vi "Chrg_Dschrg_No_cDAQ0.vi"(0 "file path (use dialog)":path, 4 "PS VISA in":refnum<visa-resource-name>, 5 "PS error in":errorcluster, 6 "DischargeCyclePath":path=path "C:/Users/ga11/Desktop/VI/results/3PtestCharge.lvm" caption="Filename", 8 "Charge/discharge":enum8{"Charge", "Discharge"}(ring), 9 "Charge/Discharge Voltage Setpoint":dbl format="%#.6g", 10 "CC or CCCV":enum16{"CC", "CCCV"}(ring), 11 "Current Setpoint":dbl format="%#.6g", 12 "Output Safety":T1, 13 "Current Cutoff":dbl) -> (18 "PS VIS resource name out":refnum<visa-resource-name>, 19 "PS error out":errorcluster)   [LabVIEW 2020]
uses:
  Drivers-Essentials/global stop1.vi
  Drivers-NHR-9200/NHR/Public/Data/Low Level/Fetch (Ave Voltage).vi
  Drivers-NHR-9200/NHR/NH Research Regenerative Test Series.lvlib
panel:
  out "error out":errorcluster
  out "Read Ave Current (A)":dbl
  out "Read Ave Voltage (V)":dbl
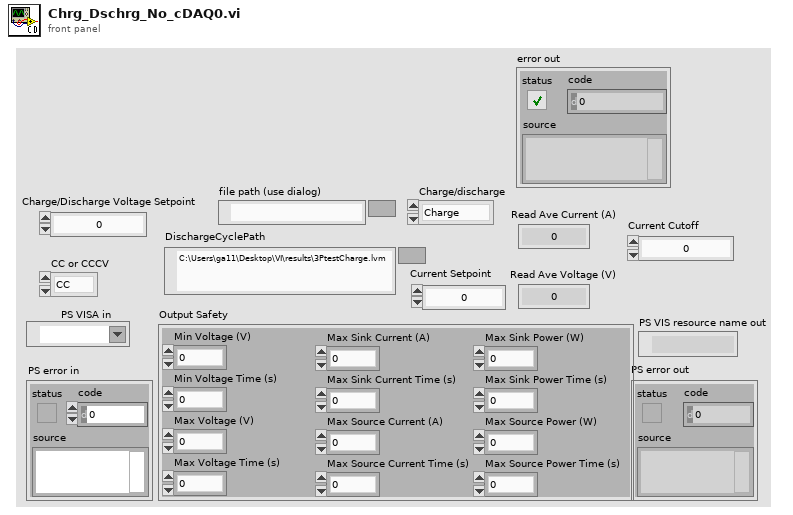
[diagram p1: front panel]
types:
  T1 = cluster{"Min Voltage (V)":dbl, "Min Voltage Time (s)":dbl, "Max Voltage (V)":dbl, "Max Voltage Time (s)":dbl, "Max Sink Current (A)":dbl, "Max Sink Current Time (s)":dbl, "Max Source Current (A)":dbl, "Max Source Current Time (s)":dbl, "Max Sink Power (W)":dbl, "Max Sink Power Time (s)":dbl, "Max Source Power (W)":dbl, "Max Source Power Time (s)":dbl}
  T2 = enum16{"open", "replace", "create", "open or create", "replace or create", "replace or create with confirmation"}
  T3 = cluster{"Voltage Enabled":bool, "Current Enabled":bool, "Power Enabled":bool, "Resistance Enabled":bool}
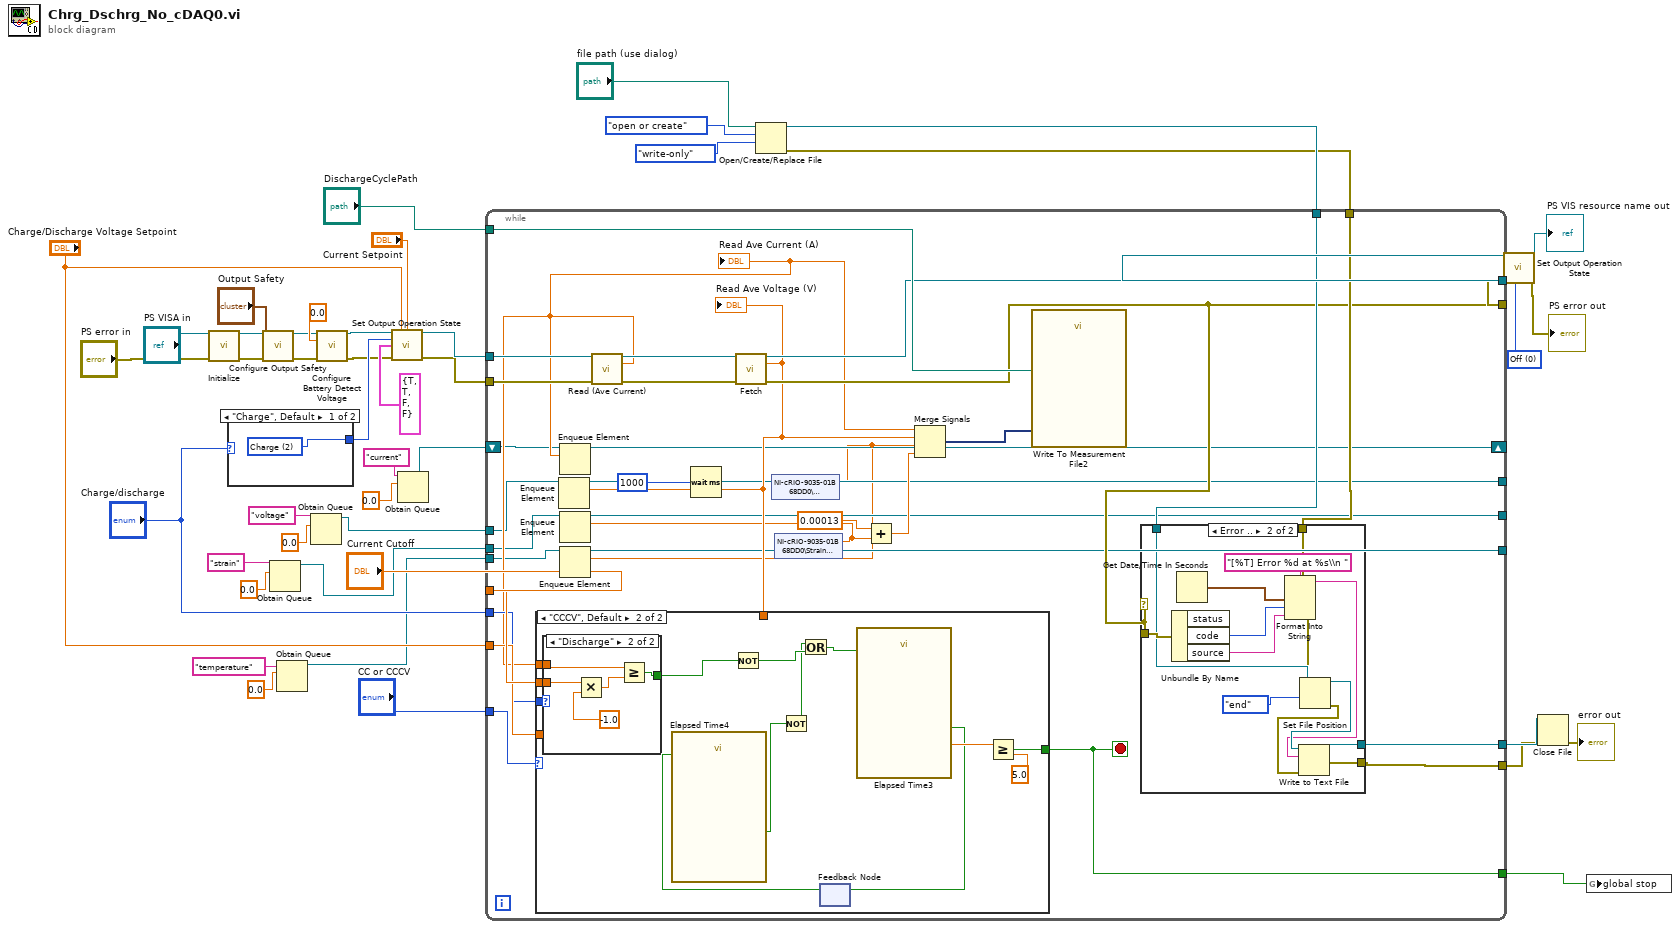
[diagram p0: block diagram]
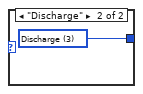
[diagram p2: hidden frame]
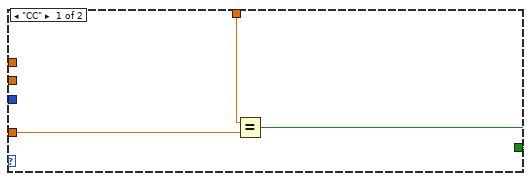
[diagram p4: hidden frame]
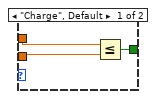
[diagram p5: hidden frame]
diagram:
  w35 = 0 items=["Off", "Standby", "Charge", "Discharge", "Battery"] ("Mode (0: Off)")
  n1 = call "Initialize.vi"("VISA resource name"="PS VISA in", "error in (no error)"="PS error in") -> ("VISA resource name out"=w26:refnum<visa-resource-name>, "error out"=w27:errorcluster)  [unwired: 12 in]
  n2 = case shown="\"Charge\", Default" "Charge/discharge" {
    tunnel: [w47 w48] -> w36
    frame "Charge", Default {
      w47 = 2 items=["Off", "Standby", "Charge", "Discharge", "Battery"] ("Mode (0: Off)")
    }
    frame "Discharge" {
      w48 = 3 items=["Off", "Standby", "Charge", "Discharge", "Battery"] ("Mode (0: Off)")
    }
  }
  n3 = call "Configure Output Safety.vi"("VISA resource name"=w26, "Output Safety"="Output Safety", "error in (no error)"=w27) -> ("VISA resource name out"=w29:refnum<visa-resource-name>, "error out"=w28:errorcluster)  [unwired: 11 in]
  n4 = Obtain Queue(name (unnamed)="strain", element data type=0.0) -> (queue out=w2:refnum<queue>)  [unwired: 3 in, 2 out]
  n5 = Obtain Queue(name (unnamed)="temperature", element data type=0.0) -> (queue out=w1:refnum<queue>)  [unwired: 3 in, 2 out]
  n6 = Obtain Queue(name (unnamed)="voltage", element data type=0.0) -> (queue out=w3:refnum<queue>)  [unwired: 3 in, 2 out]
  n7 = call "Configure Battery Detect Voltage.vi"("VISA resource name"=w29, "Battery Detect Voltage (0V)"=0.0, "error in (no error)"=w28) -> ("VISA resource name out"=w34:refnum<visa-resource-name>, "error out"=w33:errorcluster)  [unwired: 11 in]
  n8 = call "Set Output Operation State.vi"("VISA resource name"=w34, "Voltage Setpoint (0 V)"="Charge/Discharge Voltage Setpoint", "Current Setpoint (0 A)"="Current Setpoint", "Mode (0: Off)"=w36, "Enable"=T3 {"Voltage Enabled"=TRUE, "Current Enabled"=TRUE, "Power Enabled"=FALSE, "Resistance Enabled"=FALSE}, "error in (no error)"=w33) -> ("VISA resource name out"=w39:refnum<visa-resource-name>, "error out"=w38:errorcluster)  [unwired: 8 in]
  n9 = Obtain Queue(name (unnamed)="current", element data type=0.0) -> (queue out=w11:refnum<queue>)  [unwired: 3 in, 2 out]
  n10 = Open/Create/Replace File(file path (use dialog)="file path (use dialog)", operation (0:open)=T2."open or create", access (0:read/write)=enum16{"read/write", "read-only", "write-only"}."write-only") -> (refnum out=w16:refnum<file>, error out=w15:errorcluster)  [unwired: 3 in, 1 out]
  n11 = while {
    tunnel: w39 -> [w78]
    tunnel: w38 -> [w77]
    tunnel: "Current Cutoff" -> [w72]
    tunnel: "DischargeCyclePath" -> [w74]
    tunnel: [w73] -> w31
    tunnel: [w62] -> w30
    tunnel: "CC or CCCV" -> [w71]
    tunnel: "Charge/Discharge Voltage Setpoint" -> [w70]
    tunnel: "Charge/discharge" -> [w69]
    tunnel: [w66] -> w18
    tunnel: [w65] -> w17
    tunnel: w16 -> [w64]
    tunnel: w15 -> [w63]
    tunnel: [w59] -> w12
    shift-right: [w57] -> _
    shift-left: w11 -> [w60]
    tunnel: [w56] -> _
    tunnel: [w55] -> _
    tunnel: [w53] -> _
    tunnel: w3 -> [w51]
    tunnel: w2 -> [w50]
    tunnel: w1 -> [w49]
    stop <- w59 stop-if-true
    n12 = call "Read (Ave Current).vi"("VISA resource name"=w78, "error in (no error)"=w77) -> ("VISA resource name out"=w79:refnum<visa-resource-name>, "Ave Current (A)"=w61:dbl, "error out"=w80:errorcluster)  [unwired: 11 in]
    "Read Ave Current (A)" <- w61
    n13 = Enqueue Element(queue=w60, element=w61) -> (queue out=w57:refnum<queue>)  [unwired: 2 in, 2 out]
    n14 = Wait (ms)(milliseconds to wait=1000) -> ()  [unwired: 1 out]
    n15 = call-poly "Fetch.vi"("VISA resource name"=w79, "error in (no error)"=w80) -> ("VISA resource name out"=w73:refnum<visa-resource-name>, "Ave Voltage (V)"=w58:dbl, "error out"=w62:errorcluster)  [unwired: 11 in]
    "Read Ave Voltage (V)" <- w58
    n16 = case shown="\"CCCV\", Default" w71 {
      tunnel: [w97 w106] -> w59
      tunnel: w72 -> [_ w103]
      tunnel: w61 -> [_ w102]
      tunnel: w58 -> [w99 _]
      tunnel: w70 -> [w98 _]
      tunnel: w69 -> [_ w100]
      frame "CC" {
        n17 = Equal?(x=w99, y=w98) -> (x = y?=w97:bool)
      }
      frame "CCCV", Default {
        n18 = case shown="\"Discharge\"" w100 {
          tunnel: w103 -> [w114 w119]
          tunnel: w102 -> [w115 w117]
          tunnel: [w113 w116] -> w101
          frame "Charge", Default {
            n19 = Less Or Equal?(x=w115, y=w114) -> (x <= y?=w113:bool)
          }
          frame "Discharge" {
            n20 = Multiply(x=w119, y=-1.0) -> (x*y=w118:dbl)
            n21 = Greater Or Equal?(x=w117, y=w118) -> (x >= y?=w116:bool)
          }
        }
        n22 = Not(x=w101) -> (.not. x?=w112:bool)
        n23 = feedback #1() -> (w104:bool)  [unwired: 1 in]
        n24 = call "Elapsed Time4"("Reset"=w104) -> ("Time has Elapsed"=w111:bool)  [unwired: 11 in, 7 out]
        n25 = Not(x=w111) -> (.not. x?=w110:bool)
        n26 = Or(x=w110, y=w112) -> (x .or. y?=w109:bool)
        n27 = call "Elapsed Time3"("Reset"=w109) -> ("Elapsed Time (s)"=w108:dbl, "Time has Elapsed"=w105:bool)  [unwired: 11 in, 6 out]
        n28 = feedback-in #1(w105) -> ()
        n29 = Greater Or Equal?(x=w108, y=5.0) -> (x >= y?=w106:bool)
      }
    }
    n30 = Enqueue Element(queue=w51, element=w58) -> (queue out=w56:refnum<queue>)  [unwired: 2 in, 2 out]
    n31 = shared-variable "NI-cRIO-9035-01B68DD0\\Thermocouple\\TCI0"() -> (w52:dbl)  [unwired: 1 in, 1 out]
    n32 = Enqueue Element(queue=w49, element=w52) -> (queue out=w53:refnum<queue>)  [unwired: 2 in, 2 out]
    n33 = shared-variable "NI-cRIO-9035-01B68DD0\\Strain Gauge\\SGI0"() -> (w54:dbl)  [unwired: 1 in, 1 out]
    n34 = Enqueue Element(queue=w50, element=w54) -> (queue out=w55:refnum<queue>)  [unwired: 2 in, 2 out]
    n35 = Add(x=0.00013, y=w54) -> (x+y=w67:dbl)
    n36 = Merge Signals "Merge Signals"(w61, w58, w52, w67) -> (w76:dynamicdata)
    n37 = call "Write To Measurement File2"("Signals"=w76, "Filename"=w74) -> ()  [unwired: 15 in, 3 out]
    n38 = case shown="Error .." w62 {
      tunnel: w62 -> [_ w96]
      tunnel: w64 -> [w82 w94]
      tunnel: [w82 w92] -> w66
      tunnel: w63 -> [w81 w91]
      tunnel: [w81 w88] -> w65
      frame No Error {
      }
      frame Error {
        n39 = Unbundle By Name(w96) -> ("code"=w85:i32, "source"=w84:string)  [unwired: 1 out]
        n40 = Get Date/Time In Seconds() -> (seconds since 1Jan1904=w86:timestamp)
        n41 = Format Into String(format string="[%T] Error %d at %s\\n ", error in=w91, w86, w85, w84) -> (resulting string=w83:string, error out=w90:errorcluster)  [unwired: 1 in]
        n42 = Set File Position(refnum=w94, from (0:start)=enum16{"start", "end", "current"}."end", error in=w90) -> (refnum out=w93:refnum<file>, error out=w89:errorcluster)  [unwired: 1 in]
        n43 = Write to Text File(file (use dialog)=w93, text=w83, error in=w89) -> (refnum out=w92:refnum<file>, error out=w88:errorcluster)  [unwired: 1 in, 1 out]
      }
    }
  }
  n44 = call "Set Output Operation State.vi"("VISA resource name"=w31, "Mode (0: Off)"=w35, "error in (no error)"=w30) -> ("VISA resource name out"=→"PS VIS resource name out":refnum<visa-resource-name>, "error out"=→"PS error out":errorcluster)  [unwired: 11 in]
  n45 = Close File(refnum=w18, error in=w17) -> (error out=→"error out":errorcluster)  [unwired: 1 out]
  n46 = global write "global stop1.vi" "global stop"(w12) -> ()
